vi "Stop All Actors.vi"(8 "error in (no error)":errorcluster, 11 "cRIO-CO2 in":refnum<class "cRIO-CO2.lvclass">) -> (0 "error out":errorcluster, 3 "cRIO-CO2 out":refnum<class "cRIO-CO2.lvclass">)   [LabVIEW 2015, in "cRIO-Carbondioxide.lvlib" / "cRIO-CO2.lvlib" / "cRIO-CO2.lvclass"]
uses:
  cRIO-CO2.lvclass
  cRIO-CO2.lvclass/cRIO-CO2.ctl
  CO2 Actor/CO2 Actor.lvclass
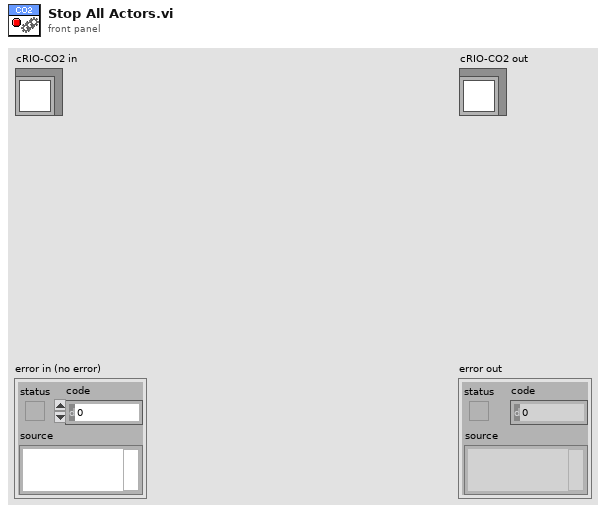
[diagram p1: front panel]
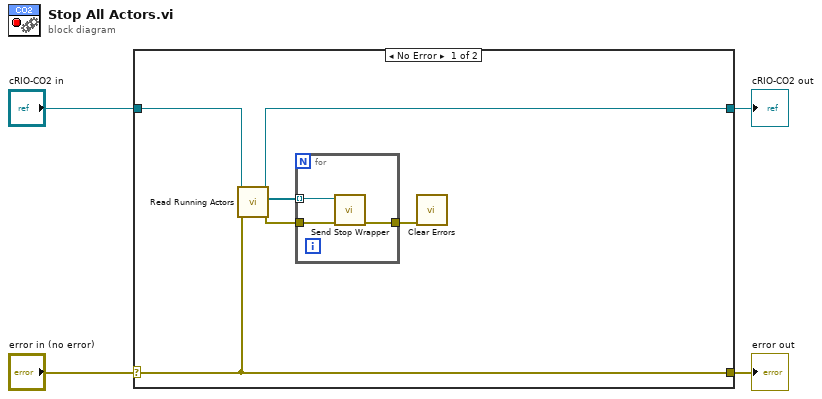
[diagram p0: block diagram]
diagram:
  n1 = case shown="No Error" "error in (no error)" {
    selector: "error in (no error)" -> [w5 w15]
    tunnel: [w5 w15] -> w3
    tunnel: [w6 w14] -> w1
    tunnel: "cRIO-CO2 in" -> [w10 w14]
    frame No Error {
      n2 = call "Read Running Actors.vi"("error in (no error)"=w5, "cRIO-CO2 in"=w10) -> ("error out"=w8:errorcluster, "Running Actors"=w9:refnum<class "CO2 Actor.lvclass">[], "cRIO-CO2 out"=w6:refnum<class "cRIO-CO2.lvclass">)  [unwired: 7 in]
      n3 = for {
        tunnel: w9 -> [w11] mode=indexing
        tunnel: w8 -> [w13]
        tunnel: [w12] -> w7
        n4 = call "Send Stop Wrapper.vi"("error in (no error)"=w13, "CO2 Actor in"=w11) -> ("error out"=w12:errorcluster)  [unwired: 8 in, 1 out]
      }
      n5 = call <vilib>:"Clear Errors.vi"("error in (no error)"=w7) -> ()  [unwired: 5 in, 2 out]
    }
    frame Error {
    }
  }
  "error out" <- w3
  "cRIO-CO2 out" <- w1
